vi "430_TCP_Query.vi"(8 "error in (no error)":errorcluster, 9 "Timeout":i32=1000, 10 "Command":string, 11 "connection ID":refnum<k5>) -> (0 "error out":errorcluster, 1 "Bytes Read":i32, 2 "Response":string, 3 "connection ID out":refnum<k5>, 4 "Bytes Written":i32)   [LabVIEW 2018]
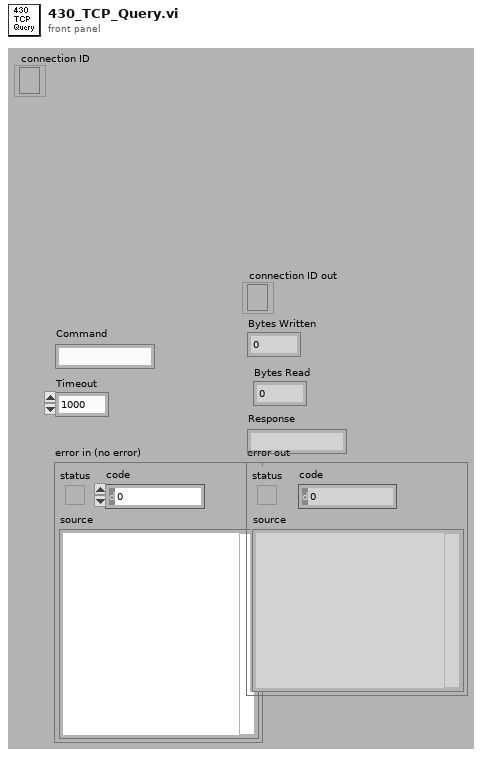
[diagram p1: front panel]
types:
  T1 = enum16{"Standard", "Buffered", "CRLF", "Immediate"}
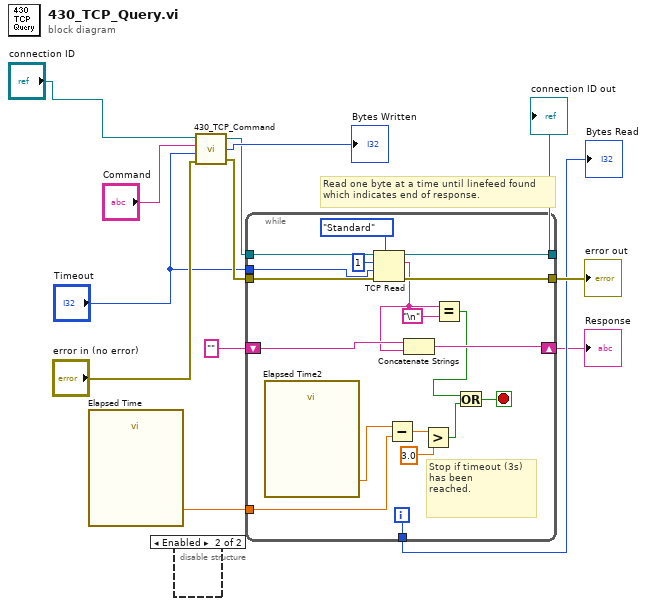
[diagram p0: block diagram]
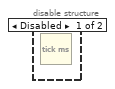
[diagram p2: hidden frame]
diagram:
  # "Read one byte at a time until linefeed found\nwhich indicates end of response."
  n1 = call "Elapsed Time"() -> ("Present (s)"=w2:dbl)  [unwired: 12 in, 7 out]
  n2 = disable-structure shown="Enabled" {
    frame Disabled {
      n3 = Tick Count (ms)() -> ()  [unwired: 1 out]
    }
    frame Enabled {
    }
  }
  n4 = call "430_TCP_Command.vi"("error in (no error)"="error in (no error)", "Timeout"="Timeout", "Command"="Command", "connection ID"="connection ID") -> ("error out"=w8:errorcluster, "bytes written"=→"Bytes Written":i32, "connection ID out"=w10:refnum<k5>)
  n5 = while {
    tunnel: w10 -> [w32]
    tunnel: [w31] -> w9
    tunnel: w8 -> [w30]
    tunnel: [w29] -> w7
    tunnel: [w28] -> w6
    shift-right: [w22] -> w3
    shift-left: "" -> [w24]
    tunnel: "Timeout" -> [w17]
    tunnel: w2 -> [w14]
    i -> [w28]
    stop <- w18 stop-if-true
    # "Stop if timeout (3s) has been\nreached."
    n6 = call "Elapsed Time2"() -> ("Present (s)"=w15:dbl)  [unwired: 12 in, 7 out]
    n7 = TCP Read(connection ID=w32, bytes to read=1, error in (no error)=w30, 7:T1."Standard" ("mode (standard)"), 9:w17) -> (connection ID out=w31:refnum<k5>, data out=w23:string, error out=w29:errorcluster)
    n8 = Subtract(x=w15, y=w14) -> (x-y=w21:dbl)
    n9 = Concatenate Strings(w24, w23) -> (w22:string)
    n10 = Greater?(x=w21, y=3.0) -> (0:w20:bool)
    n11 = Equal?(x=w23, y="\n") -> (x = y?=w19:bool)
    n12 = Or(x=w19, y=w20) -> (x .or. y?=w18:bool)
  }
  "error out" <- w7
  "Bytes Read" <- w6
  "Response" <- w3
  "connection ID out" <- w9
